vi "list and create PG alarms table_1.vi"(8 "error in":errorcluster, 10 "table name":string, 11 "conn":u32) -> (0 "error out":errorcluster, 3 "conn_out":u32)   [LabVIEW 2019, in "PostgreSQL.lvlib"]
uses:
  PostgreSQL.lvlib
  PostgreSQL2LabVIEW/libpqlv/src/PQresultErrorMessage.vi
  PostgreSQL2LabVIEW/libpqUtility/src/PQclear.vi
  PostgreSQL2LabVIEW/libpqlv/src/PQsendQuery.vi
  PostgreSQL2LabVIEW/libpqlv/src/PQgetResult.vi
  PostgreSQL2LabVIEW/libpqlv/src/PQresultStatus.vi
  PostgreSQL2LabVIEW/libpqUtility/src/PQgetColumn.vi
  PostgreSQL2LabVIEW/libpqlv/src/PQclear.vi
  PostgreSQL2LabVIEW/libpqUtility/src/PQfetchTables.vi
  PostgreSQL2LabVIEW/libpqlv/src/PQgetvalue.vi
  PostgreSQL2LabVIEW/libpqlv/src/PQntuples.vi
  PostgreSQL2LabVIEW/libpqUtility/libpqutility.lvlib
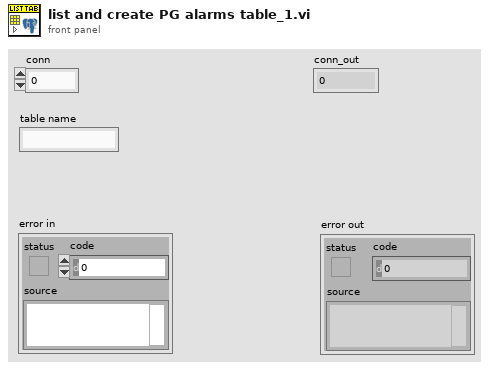
[diagram p1: front panel]
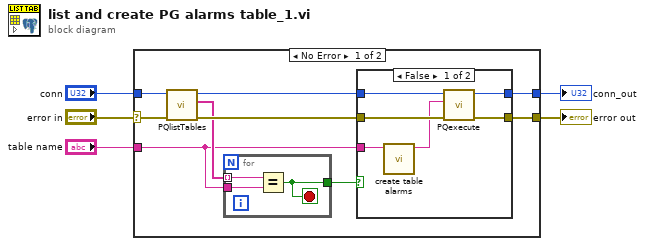
[diagram p0: block diagram]
diagram:
  n1 = case shown="No Error" "error in" {
    selector: "error in" -> [w11 w27]
    tunnel: "conn" -> [w8 w26]
    tunnel: [w14 w26] -> w3
    tunnel: [w13 w27] -> w2
    tunnel: "table name" -> [w6 _]
    frame No Error {
      n2 = call "PQlistTables.vi"("error in"=w11, "conn"=w8) -> ("error out"=w10:errorcluster, "Data"=w7:string[], "conn_out"=w9:u32)  [unwired: 7 in]
      n3 = for {
        tunnel: w6 -> [w16]
        tunnel: w7 -> [w17] mode=indexing
        tunnel: [w15] -> w12
        stop <- w15 stop-if-true
        n4 = Equal?(x=w17, y=w16) -> (x = y?=w15:bool)
      }
      n5 = case shown="False" w12 {
        tunnel: w9 -> [w23 w25]
        tunnel: [w21 w25] -> w14
        tunnel: w10 -> [w22 w24]
        tunnel: [w20 w24] -> w13
        tunnel: w6 -> [w18 _]
        frame False {
          n6 = call "create table alarms.vi"("table name"=w18) -> ("create table parameters"=w19:string)  [unwired: 10 in]
          n7 = call "PQexecute.vi"("error in"=w22, "SQL querry"=w19, "conn"=w23) -> ("error out"=w20:errorcluster, "conn_out"=w21:u32)  [unwired: 7 in]
        }
        frame True {
        }
      }
    }
    frame Error {
    }
  }
  "conn_out" <- w3
  "error out" <- w2
